vi "Move.vi"(7 "VI Ref":refnum<vi>, 8 "Error":errorcluster, 11 "DecFrame_FP":refnum<class "DecFrame_FP.lvclass">) -> (0 "Error Out":errorcluster, 3 "DecFrame_FP Out":refnum<class "DecFrame_FP.lvclass">, 5 "VI Out":refnum<vi>)   [LabVIEW 2016, in "DecFrame_FP.lvclass"]
uses:
  DecFrame_FP.lvclass
  E:/~Data/FRC/Magic Trident/Code/UI LED Build file Interface/Utility/Universal Utility/FP/FPClass/(FP)/(FP).lvclass
  DecFrame_FP.lvclass/DecFrame_FP.ctl
  (FPPos)/Frame_FPPos/Frame_FPPos.lvclass
  (FP).lvclass
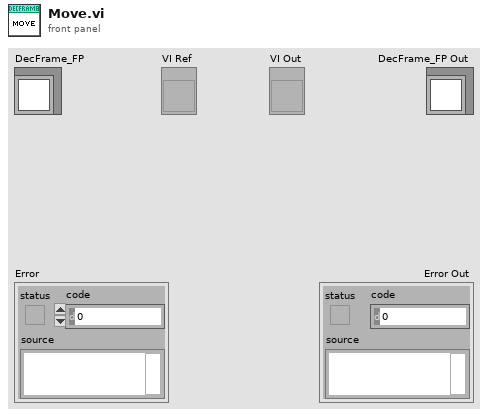
[diagram p1: front panel]
types:
  T1 = typedef "LVRectTypeDef.ctl" = cluster{"Left":i16, "Top":i16, "Right":i16, "Bottom":i16}
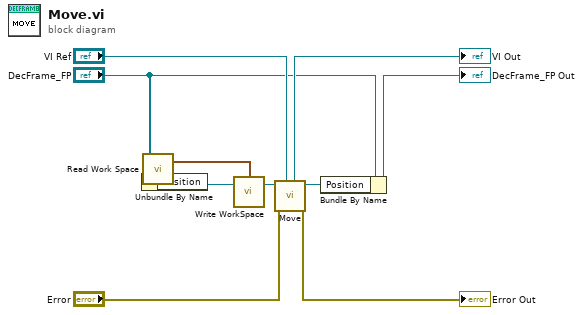
[diagram p0: block diagram]
diagram:
  n1 = Unbundle By Name("DecFrame_FP") -> ("Position"=w6:refnum<class "Frame_FPPos.lvclass">)
  n2 = call "Read Work Space.vi"("(FP)"="DecFrame_FP") -> ("WkSpace Out"=w4:T1)  [unwired: 2 in]
  n3 = call "Write WorkSpace.vi"("(FPPos)"=w6, "WkSpace"=w4) -> ("(FPPos) Out"=w5:refnum<class "Frame_FPPos.lvclass">)  [unwired: 3 in]
  n4 = call-dynamic "Move.vi"("VI"="VI Ref", "Error"="Error", "(FPPos)"=w5) -> ("Error Out"=→"Error Out":errorcluster, "(FPPos) Out"=w1:refnum<class "Frame_FPPos.lvclass">, "VI Out"=→"VI Out":refnum<vi>)  [unwired: 6 in]
  n5 = Bundle By Name(cluster="DecFrame_FP", "Position"=w1) -> (→"DecFrame_FP Out":refnum<class "DecFrame_FP.lvclass">)
